vi "Correct Exctinction.vi"(8 "error in":errorcluster, 10 "refExt":sgl, 11 "CRDS Cell Data in":refnum<class "CRDS Cell Data.lvclass">) -> (0 "error out":errorcluster, 3 "CRDS Cell Data out":refnum<class "CRDS Cell Data.lvclass">)   [LabVIEW 2016, in "CRDS Lib.lvlib" / "CRDS Cell Data.lvclass"]
doc: "Remove gas phase extinction from the non-reference channels (i.e. those that are sampling aerosol, the dry and humidified channels)."
uses:
  CRDS Cell Data.lvclass
  CRDS Cell Data.lvclass/CRDS Cell Data.ctl
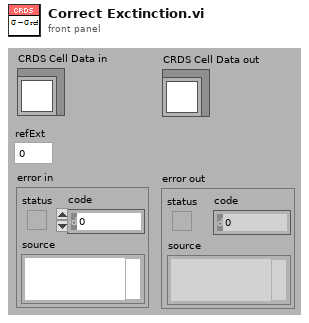
[diagram p1: front panel]
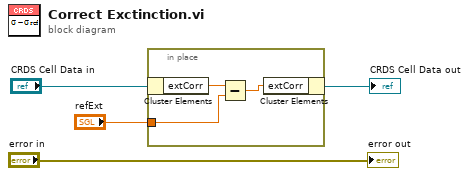
[diagram p0: block diagram]
diagram:
  n1 = in-place {
    in-place-border: "refExt" -> [w6]
    n2 = in-place-cluster #1("CRDS Cell Data in") -> ("extCorr"=w7:sgl)
    n3 = Subtract(x=w7, y=w6) -> (x-y=w5:sgl)
    n4 = in-place-cluster #1("extCorr"=w5) -> (→"CRDS Cell Data out":refnum<class "CRDS Cell Data.lvclass">)
  }
  "error out" <- "error in"
